vi "convert_2DimString_to_Plot.vi"(8 "error in (no error)":errorcluster, 10 "string data in":string[][](array[string])) -> (0 "error out":errorcluster, 2 "Plot Data":cluster{dbl, dbl, "flag":u8}[](array[cluster]))   [LabVIEW 2015]
doc: "converts an 2-dim array of strings to a 1-dim array of clusters of x-y-data (data or a plot).\nThis can be used to convert:\nAnalysis Data\nScan Data"
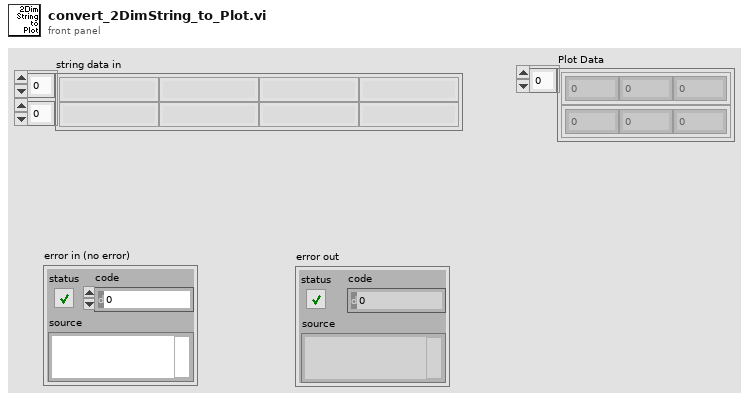
[diagram p1: front panel]
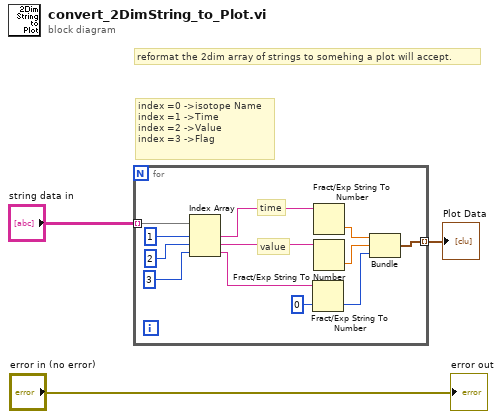
[diagram p0: block diagram]
diagram:
  # "reformat the 2dim array of strings to somehing a plot will accept."
  # "index =0 ->isotope Name\nindex =1 ->Time\nindex =2 ->Value\nindex =3 ->Flag"
  n1 = for {
    tunnel: "string data in" -> [w15] mode=indexing
    tunnel: [w8] -> w2 mode=indexing
    # "value"
    # "time"
    n2 = Index Array(array=w15, index #1=1 ("index"), index #2=2 ("index"), index #3=3 ("index")) -> (element #1=w12:string, element #2=w11:string, element #3=w6:string)
    n3 = Fract/Exp String To Number(string=w6, default (0 dbl)=u8 0) -> (number=w4:u8)  [unwired: 2 in, 1 out]
    n4 = Fract/Exp String To Number(string=w12) -> (number=w10:dbl)  [unwired: 3 in, 1 out]
    n5 = Fract/Exp String To Number(string=w11) -> (number=w9:dbl)  [unwired: 3 in, 1 out]
    n6 = Bundle(w10, w9, w4) -> (w8:cluster{dbl, dbl, u8})  [unwired: 1 in]
  }
  "Plot Data" <- w2
  "error out" <- "error in (no error)"
